vi "SendDSProtocol.vi"(7 "Send":bool, 9 "Initialize":bool, 10 "DS old":T1={"type"="Driverstation", "device"="", "name"="", "data"={">enabled"=FALSE, ">autonomous"=FALSE, ">test"=FALSE, ">estop"=FALSE, ">fms"=FALSE, ">ds"=FALSE, "<match_time"=0.0, ">station"="", ">game_data"=""}}, 11 "DS new":T1={"type"="Driverstation", "device"="", "name"="", "data"={">enabled"=FALSE, ">autonomous"=FALSE, ">test"=FALSE, ">estop"=FALSE, ">fms"=FALSE, ">ds"=FALSE, "<match_time"=0.0, ">station"="", ">game_data"=""}}) -> ()   [LabVIEW 2019]
uses:
  DS proto.ctl
  DS data proto.ctl
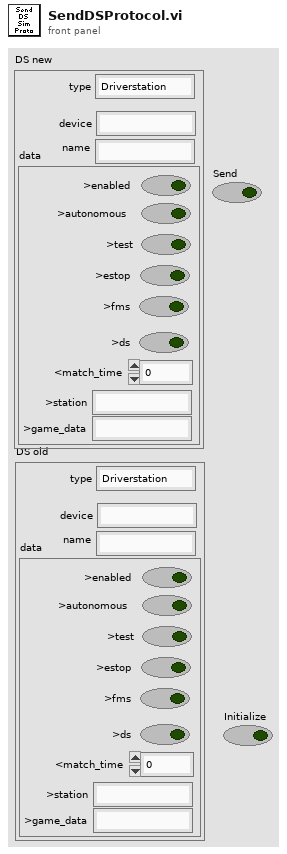
[diagram p1: front panel]
types:
  T1 = typedef "DS proto.ctl" = cluster{"type":string, "device":string, "name":string, "data":T2}
  T2 = typedef "DS data proto.ctl" = cluster{">enabled":bool, ">autonomous":bool, ">test":bool, ">estop":bool, ">fms":bool, ">ds":bool, "<match_time":dbl, ">station":string, ">game_data":string}
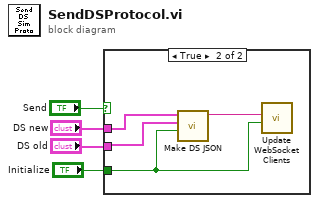
[diagram p0: block diagram]
diagram:
  n1 = case shown="True" "Send" {
    tunnel: "DS new" -> [_ w8]
    tunnel: "DS old" -> [_ w6]
    tunnel: "Initialize" -> [_ w5]
    frame False {
    }
    frame True {
      n2 = call "Make DS JSON.vi"("Force"=w5, "Driverstation prev"=w6, "Driverstation new"=w8) -> ("delta JSON"=w7:string)  [unwired: 8 in]
      n3 = call "Update WebSocket Clients.vi"("Initialize"=w5, "delta JSON"=w7) -> ()  [unwired: 10 in]
    }
  }
